vi "CreateActionQueues.vi"(8 "Error In":errorcluster) -> (0 "Error Out":errorcluster, 3 "Action Queues":T1)   [LabVIEW 2012]
uses:
  ActionQueues.ctl
  UIActionQueueElement.ctl
  UIAction.ctl
  HardwareActionQueueElement.ctl
  HardwareAction.ctl
  LogActionQueueElement.ctl
  LogAction.ctl
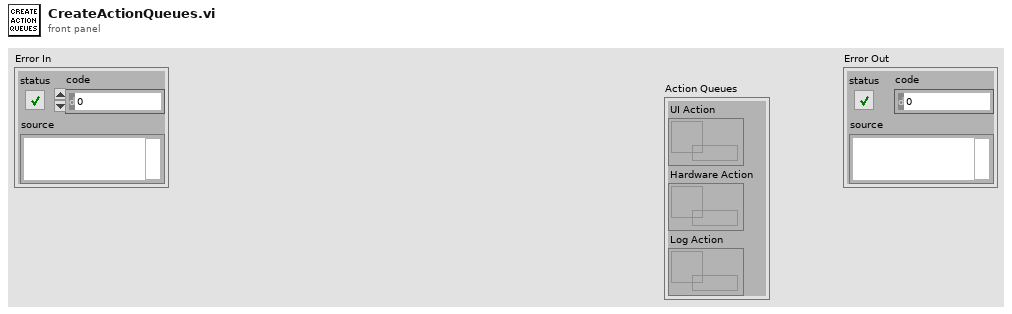
[diagram p1: front panel]
types:
  T1 = typedef "ActionQueues.ctl" = cluster{"UI Action":refnum<queue>, "Hardware Action":refnum<queue>, "Log Action":refnum<queue>}
  T2 = typedef "LogActionQueueElement.ctl" = cluster{"Action":T3, "Data":variant}
  T3 = typedef "LogAction.ctl" = enum16{"Initialize", "Start", "Arm", "Create", "Write", "Close", "Rearm", "Stop", "Error", "Shutdown"}
  T4 = typedef "HardwareActionQueueElement.ctl" = cluster{"Action":T5, "Data":variant}
  T5 = typedef "HardwareAction.ctl" = enum16{"Initialize", "Start", "Run", "Stop", "Error", "Shutdown"}
  T6 = typedef "UIActionQueueElement.ctl" = cluster{"Action":T7, "Data":variant}
  T7 = typedef "UIAction.ctl" = enum16{"Initialize", "Configure Trigger", "Configure Measure", "Configure Source", "Configure DUT", "Configure Log", "Configure Open", "Configure Save", "Configure Reset", "Hardware Start", "Hardware Started", "Hardware Stop", "Hardware Stopped", "Log Arm", "Log Start", "Log Started", "Log Stop", "Log Stopped", "Error", "Shutdown"}
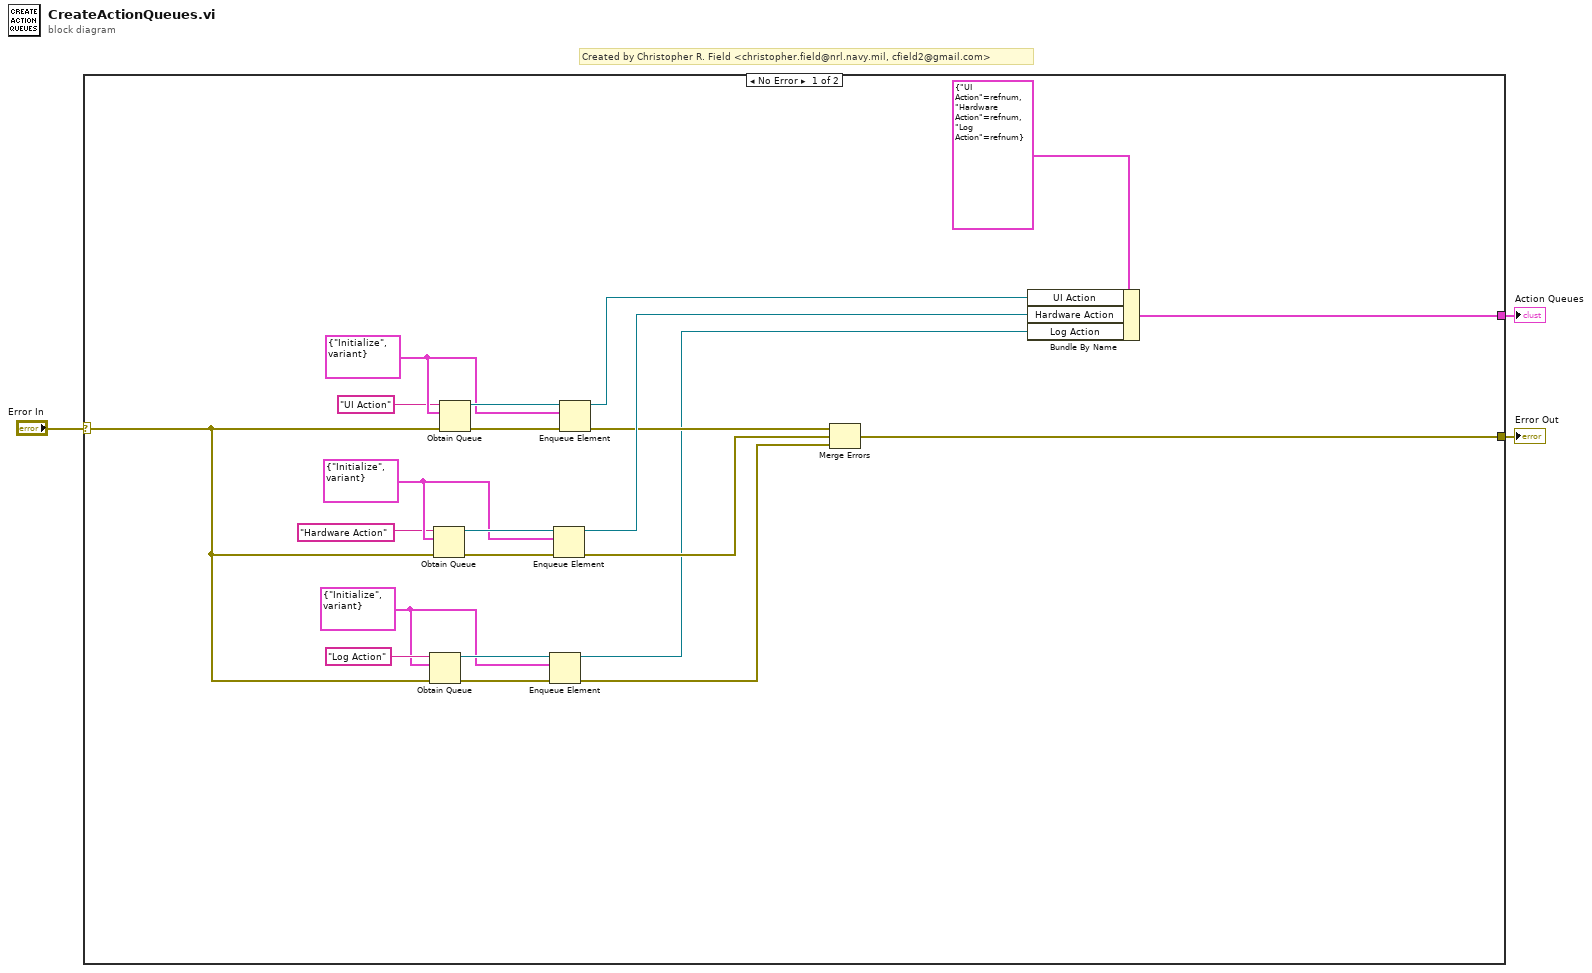
[diagram p0: block diagram]
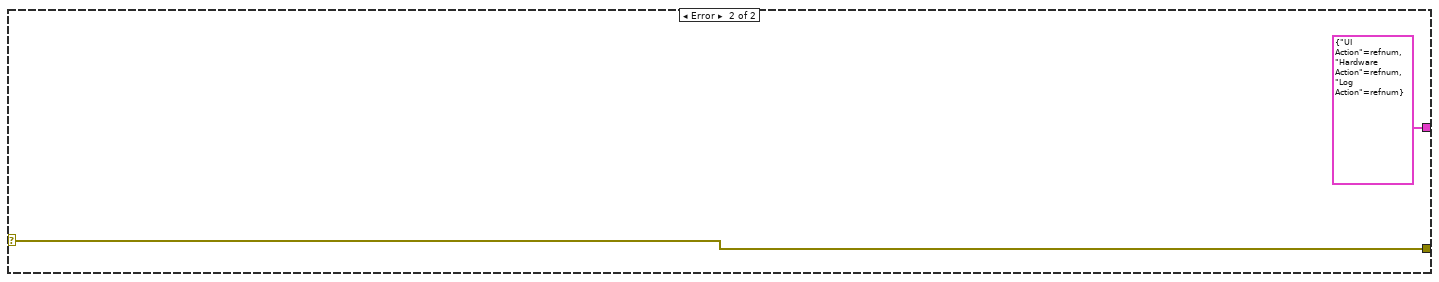
[diagram p2: hidden frame]
diagram:
  # "Created by Christopher R. Field <christopher.field@nrl.navy.mil, cfield2@gmail.com>"
  n1 = case shown="No Error" "Error In" {
    selector: "Error In" -> [w9 w27]
    tunnel: [w11 w27] -> w2
    tunnel: [w19 T1 {"UI Action"=refnum, "Hardware Action"=refnum, "Log Action"=refnum} ("Action Queues")] -> w1
    frame No Error {
      w5 = T2 {"Action"=enum."Initialize", "Data"=variant} ("Log Action Queue Element")
      w16 = T4 {"Action"=enum."Initialize", "Data"=variant} ("Hardware Action Queue Element")
      w23 = T6 {"Action"=enum."Initialize", "Data"=variant} ("UI Action Queue Element")
      n2 = Obtain Queue(name (unnamed)="Log Action", element data type=w5, error in (no error)=w9) -> (queue out=w7:refnum<queue>, error out=w8:errorcluster)  [unwired: 2 in, 1 out]
      n3 = Obtain Queue(name (unnamed)="Hardware Action", element data type=w16, error in (no error)=w9) -> (queue out=w18:refnum<queue>, error out=w17:errorcluster)  [unwired: 2 in, 1 out]
      n4 = Obtain Queue(name (unnamed)="UI Action", element data type=w23, error in (no error)=w9) -> (queue out=w25:refnum<queue>, error out=w24:errorcluster)  [unwired: 2 in, 1 out]
      n5 = Enqueue Element(queue=w7, element=w5, error in (no error)=w8) -> (queue out=w4:refnum<queue>, error out=w6:errorcluster)  [unwired: 1 in, 1 out]
      n6 = Enqueue Element(queue=w18, element=w16, error in (no error)=w17) -> (queue out=w14:refnum<queue>, error out=w12:errorcluster)  [unwired: 1 in, 1 out]
      n7 = Enqueue Element(queue=w25, element=w23, error in (no error)=w24) -> (queue out=w20:refnum<queue>, error out=w13:errorcluster)  [unwired: 1 in, 1 out]
      n8 = Merge Errors(w13, w12, w6) -> (w11:errorcluster)
      n9 = Bundle By Name(cluster=T1 {"UI Action"=refnum, "Hardware Action"=refnum, "Log Action"=refnum} ("Action Queues"), "UI Action"=w20, "Hardware Action"=w14, "Log Action"=w4) -> (w19:T1)
    }
    frame Error {
    }
  }
  "Error Out" <- w2
  "Action Queues" <- w1
